vi "Save_enable.vi"(8 "error in (no error)":errorcluster, 10 "Save?":bool, 11 "GUI_Actor in":refnum<class "GUI_Actor.lvclass">) -> (0 "error out":errorcluster, 3 "GUI_Actor out":refnum<class "GUI_Actor.lvclass">)   [LabVIEW 2019, in "GUI_Actor.lvlib" / "GUI_Actor.lvclass"]
uses:
  GUI_Actor.lvclass
  GUI_Actor.lvclass/GUI_Actor.ctl
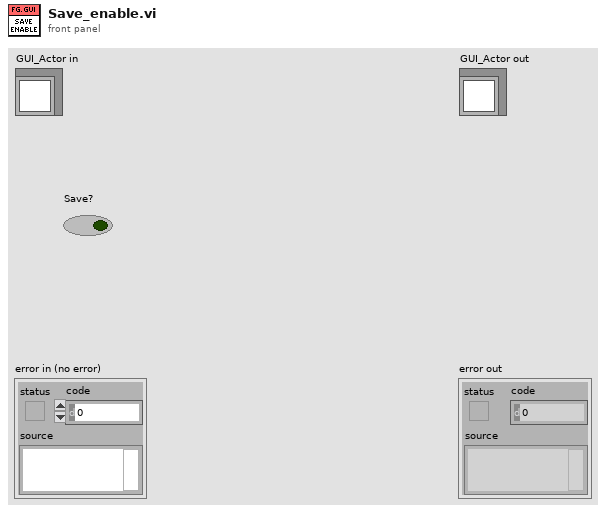
[diagram p1: front panel]
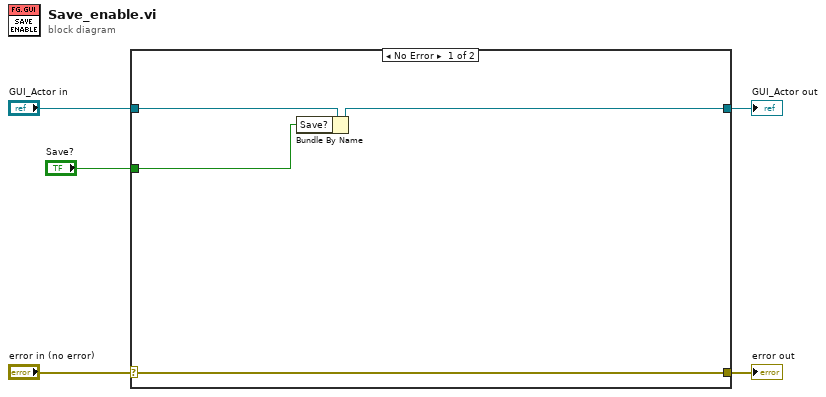
[diagram p0: block diagram]
diagram:
  n1 = case shown="No Error" "error in (no error)" {
    selector: "error in (no error)" -> [w8 w11]
    tunnel: [w8 w11] -> w4
    tunnel: [w7 w10] -> w2
    tunnel: "GUI_Actor in" -> [w9 w10]
    tunnel: "Save?" -> [w6 _]
    frame No Error {
      n2 = Bundle By Name(cluster=w9, "Save?"=w6) -> (w7:refnum<class "GUI_Actor.lvclass">)
    }
    frame Error {
    }
  }
  "error out" <- w4
  "GUI_Actor out" <- w2
